vi "Update TX Slot Display.vi"(8 "error in":errorcluster, 9 "Location":cluster{"X":i32, "Y":i32}, 10 "Button":i32, 11 "UI Actor in":refnum<class "UI Actor.lvclass">) -> (0 "error out":errorcluster, 3 "UI Actor out":refnum<class "UI Actor.lvclass">)   [LabVIEW 2024, in "UI Actor.lvlib" / "UI Actor.lvclass"]
uses:
  UI Actor.lvclass
  UI Actor.lvclass/UI Actor.ctl
  Controls/TX Communication Parameter.ctl
  320aeeb9-ea85-43b7-8258-4ae750d7a996.vi
  <vilib>/JDP Science/JSONtext/Find Item.vi
  <vilib>/JDP Science/JSONtext/Next JSON Value.vi
  <vilib>/JDP Science/JSONtext/String Subset.vi
  <vilib>/JDP Science/JSONtext/Parsing/Advance past next JSON Value (inlined COPY).vi
  <vilib>/JDP Science/JSONtext/Parsing/Advance past whitespace.vi
  <vilib>/JDP Science/JSONtext/Parsing/Advance past String.vi
  <vilib>/JDP Science/JSONtext/Parsing/Advance past Number.vi
  <vilib>/JDP Science/JSONtext/Parsing/Advance past Line Ending.vi
  PDO Grid/PDO Grid.lvclass
  <vilib>/JDP Science/JSONtext/Parsing/Parse Full Path or Item Name.vi
  <vilib>/JDP Science/JSONtext/Parsing/Advance past Array.vi
  <vilib>/JDP Science/JSONtext/Parsing/Advance past Object.vi
  <vilib>/JDP Science/JSONtext/support/Error Cluster From Code.vi
  <vilib>/JDP Science/JSONtext/Offset/Find Item Locations by Path.vi
  <vilib>/JDP Science/JSONtext/JSON text to Variant.vi
  <vilib>/JDP Science/JSONtext/LVClass Serializer/JSONtext LVClass Serializer.lvclass
  Sourcegrid-LabVIEW/source/Cells/Cell/Cell.lvclass
  Sourcegrid-LabVIEW/source/Grid/SourceGrid.lvclass
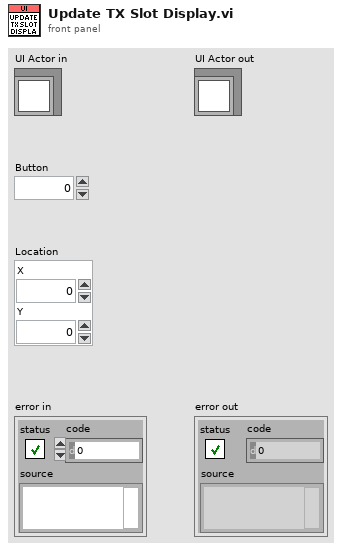
[diagram p1: front panel]
types:
  T1 = typedef "UI Actor.lvlib/UI Actor.lvclass/TX Communication Parameter.ctl" = cluster{"Communication":u16, "Mapping":u16, "COB":u32, "Type":u8, "Inhibit":u16, "Event Timer":u16, "Sync Start":u8}
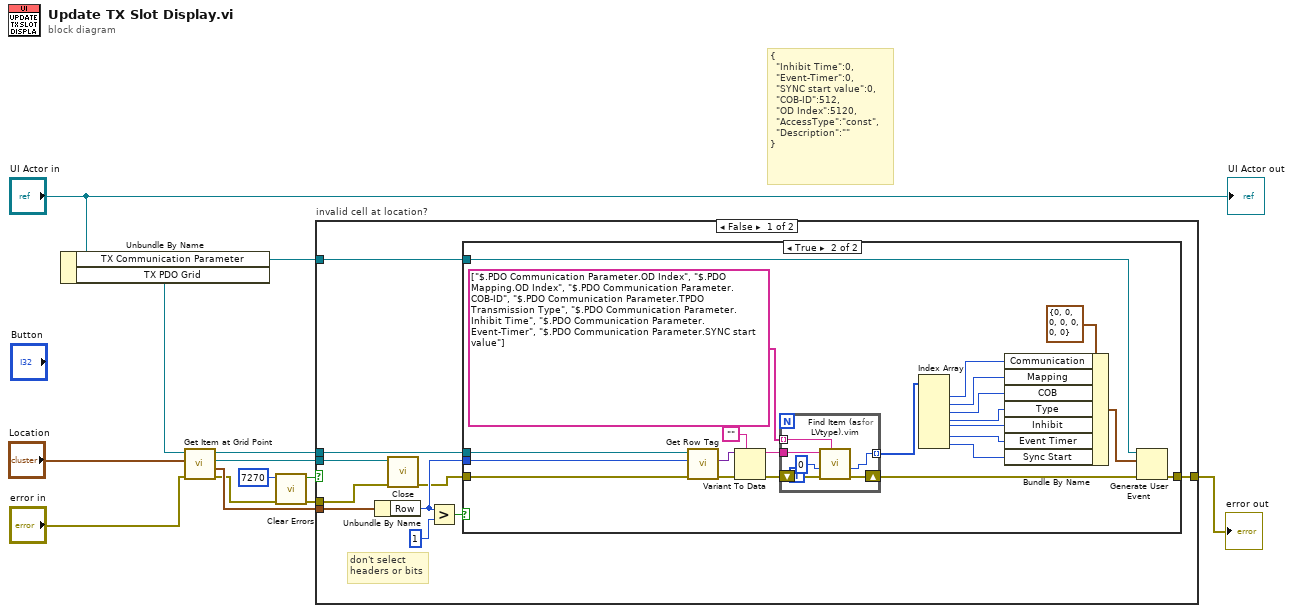
[diagram p0: block diagram]
diagram:
  # "{\n  \"Inhibit Time\":0,\n  \"Event-Timer\":0,\n  \"SYNC start value\":0,\n  \"COB-ID\":512,\n  \"OD Index\":5120,\n  \"AccessType\":\"const\",\n  \"Description\":\"\"\n}"
  n1 = Unbundle By Name("UI Actor in") -> ("TX Communication Parameter"=w4:refnum<user-event>, "TX PDO Grid"=w12:refnum<class "PDO Grid.lvclass">)
  n2 = call "Get Item at Grid Point.vi"("error in"="error in", "Location"="Location", "SourceGrid in"=w12) -> ("error out"=w8:errorcluster, "Cell Position"=w9:cluster{"Row":i32, "Column":i32}, "Cell out"=w5:refnum<class "Cell.lvclass">, "SourceGrid out"=w7:refnum<class "PDO Grid.lvclass">)  [unwired: 5 in]
  n3 = call <vilib>:"Clear Errors.vi"("error in (no error)"=w8, "specific error code to clear (0: all)"=7270) -> ("error out"=w2:errorcluster, "specific error cleared?"=w1:bool)  [unwired: 4 in]
  n4 = case "invalid cell at location?" shown="False" w1 {
    tunnel: w9 -> [w23 _]
    tunnel: w2 -> [w21 w53]
    tunnel: w7 -> [w20 _]
    tunnel: [w19 w53] -> w6
    tunnel: w5 -> [w15 _]
    tunnel: w4 -> [w14 _]
    frame False {
      # "don't select\nheaders or bits"
      n5 = Unbundle By Name(w23) -> ("Row"=w18:i32)
      n6 = call-dynamic "Close.vi"("error in"=w21, "Cell in"=w15) -> ("error out"=w16:errorcluster)  [unwired: 8 in, 1 out]
      n7 = Greater?(x=w18, y=1) -> (0:w17:bool)
      n8 = case shown="True" w17 {
        tunnel: w16 -> [w24 w46]
        tunnel: w20 -> [_ w45]
        tunnel: [w24 w36] -> w19
        tunnel: w18 -> [_ w43]
        tunnel: w14 -> [_ w35]
        frame False {
        }
        frame True {
          n9 = call "Get Row Tag.vi"("error in"=w46, "Row Index"=w43, "SourceGrid in"=w45) -> ("error out"=w44:errorcluster, "object"=w42:variant)  [unwired: 6 in, 1 out]
          n10 = Variant To Data(error in=w44, type="", Variant=w42) -> (data=w40:string, error out=w38:errorcluster)
          n11 = for {
            tunnel: w40 -> [w49]
            tunnel: string[] ["$.PDO Communication Parameter.OD Index", "$.PDO Mapping.OD Index", "$.PDO Communication Parameter.COB-ID", "$.PDO Communication Parameter.TPDO Transmission Type", "$.PDO Communication Parameter.Inhibit Time", "$.PDO Communication Parameter.Event-Timer", "$.PDO Communication Parameter.SYNC start value"] -> [w52] mode=indexing
            shift-right: [w50] -> w37
            shift-left: w38 -> [w51]
            tunnel: [w48] -> w32 mode=indexing
            n12 = call "Find Item (as LVtype).vim"("$Path or Item Name"=w52, "error in (no error)"=w51, "Data Type and Default Value"=u32 0, "JSON"=w49) -> ("error out"=w50:errorcluster, "Data"=w48:u32)  [unwired: 4 in, 2 out]
          }
          n13 = Index Array(array=w32) -> (element #1=w31:u32, element #2=w30:u32, element #3=w29:u32, element #4=w28:u32, element #5=w27:u32, element #6=w26:u32, element #7=w25:u32)  [unwired: 7 in]
          n14 = Bundle By Name(cluster=T1 {"Communication"=0, "Mapping"=0, "COB"=0, "Type"=0, "Inhibit"=0, "Event Timer"=0, "Sync Start"=0} ("event data"), "Communication"=w31, "Mapping"=w30, "COB"=w29, "Type"=w28, "Inhibit"=w27, "Event Timer"=w26, "Sync Start"=w25) -> (w33:T1)
          n15 = Generate User Event(user event=w35, event data cluster=w33, error in=w37) -> (error out=w36:errorcluster)  [unwired: 1 in, 1 out]
        }
      }
    }
    frame True {
    }
  }
  "error out" <- w6
  "UI Actor out" <- "UI Actor in"
